vi "Unit Test Preserve wired non-serialized data (Less-Specific) True.vi"() -> ()   [LabVIEW 2019, in "Sports Unit Tests.lvclass"]
uses:
  Sports Unit Tests.lvclass
  <userlib>/Blue Origin/BlueSerialization/BlueSerializer/DeserializeOptions.ctl
  <userlib>/Blue Origin/BlueSerialization/BlueSerializer/DeserializeSlicingOptions.ctl
  <userlib>/Blue Origin/BlueSerialization/BlueSerializer/DeserializeMutationOptions.ctl
  <userlib>/Blue Origin/BlueSerialization/BlueSerializer/DeserializePreservationOptions.ctl
  <userlib>/Blue Origin/BlueSerialization/BlueSerializer/PreserveNonWiredDataOption.ctl
  Classes/The Waterboy/The Waterboy.lvclass
  C:/DSCE code/Serialization/blueserializationdemo/Test/Sports/Classes/Human/Human.lvclass
  C:/DSCE code/Serialization/blueserializationdemo/Test/Sports/Classes/Sports Player/Sports Player.lvclass
  C:/DSCE code/Serialization/blueserializationdemo/Test/Sports/Classes/Golf Player/Golf Player.lvclass
  C:/DSCE code/Serialization/blueserializationdemo/Test/Sports/Classes/Adam Sandler/Adam Sandler.lvclass
  Classes/Adam Sandler/Adam Sandler.lvclass
  Classes/Human/Human.lvclass/Human.ctl
  Classes/Sports Player/Sports Player.lvclass/Sports Player.ctl
  Classes/Golf Player/Golf Player.lvclass/Golf Player.ctl
  Classes/Adam Sandler/Adam Sandler.lvclass/Adam Sandler.ctl
  Classes/Human/Write Age (years).vi
  Classes/Human/Write alive_.vi
  Classes/Human/Write Height (ft).vi
  Classes/Human/Write Name.vi
  Classes/Sports Player/Write Earnings (dollars).vi
  Classes/Sports Player/Write Professional_.vi
  Classes/Sports Player/Write Sponsor.vi
  Classes/Golf Player/Write # holes in one.vi
  Classes/Golf Player/Write League.vi
  Classes/Golf Player/Write longest drive (ft).vi
  Classes/Adam Sandler/Write Movie Name.vi
  Classes/Adam Sandler/Write Private number.vi
  Classes/Adam Sandler/Write Secret phrase.vi
  Classes/Adam Sandler/Read Secret phrase.vi
  <vilib>/Utility/error.llb/Clear Errors.vi
  <vilib>/addons/_JKI Toolkits/Caraya/classes/Test/Define Test.vi
  <vilib>/addons/_JKI Toolkits/Caraya/classes/Assert/Assert Equal Value_Variant.vi
  <vilib>/addons/_JKI Toolkits/Caraya/classes/Assert/Assert Not Error.vi
  <vilib>/addons/_JKI Toolkits/Caraya/classes/Assert/Assert.lvclass
  <userlib>/Blue Origin/BlueSerialization/BlueSerializer/BlueSerializer.lvclass
panel:
  out "Table":string[][](table)
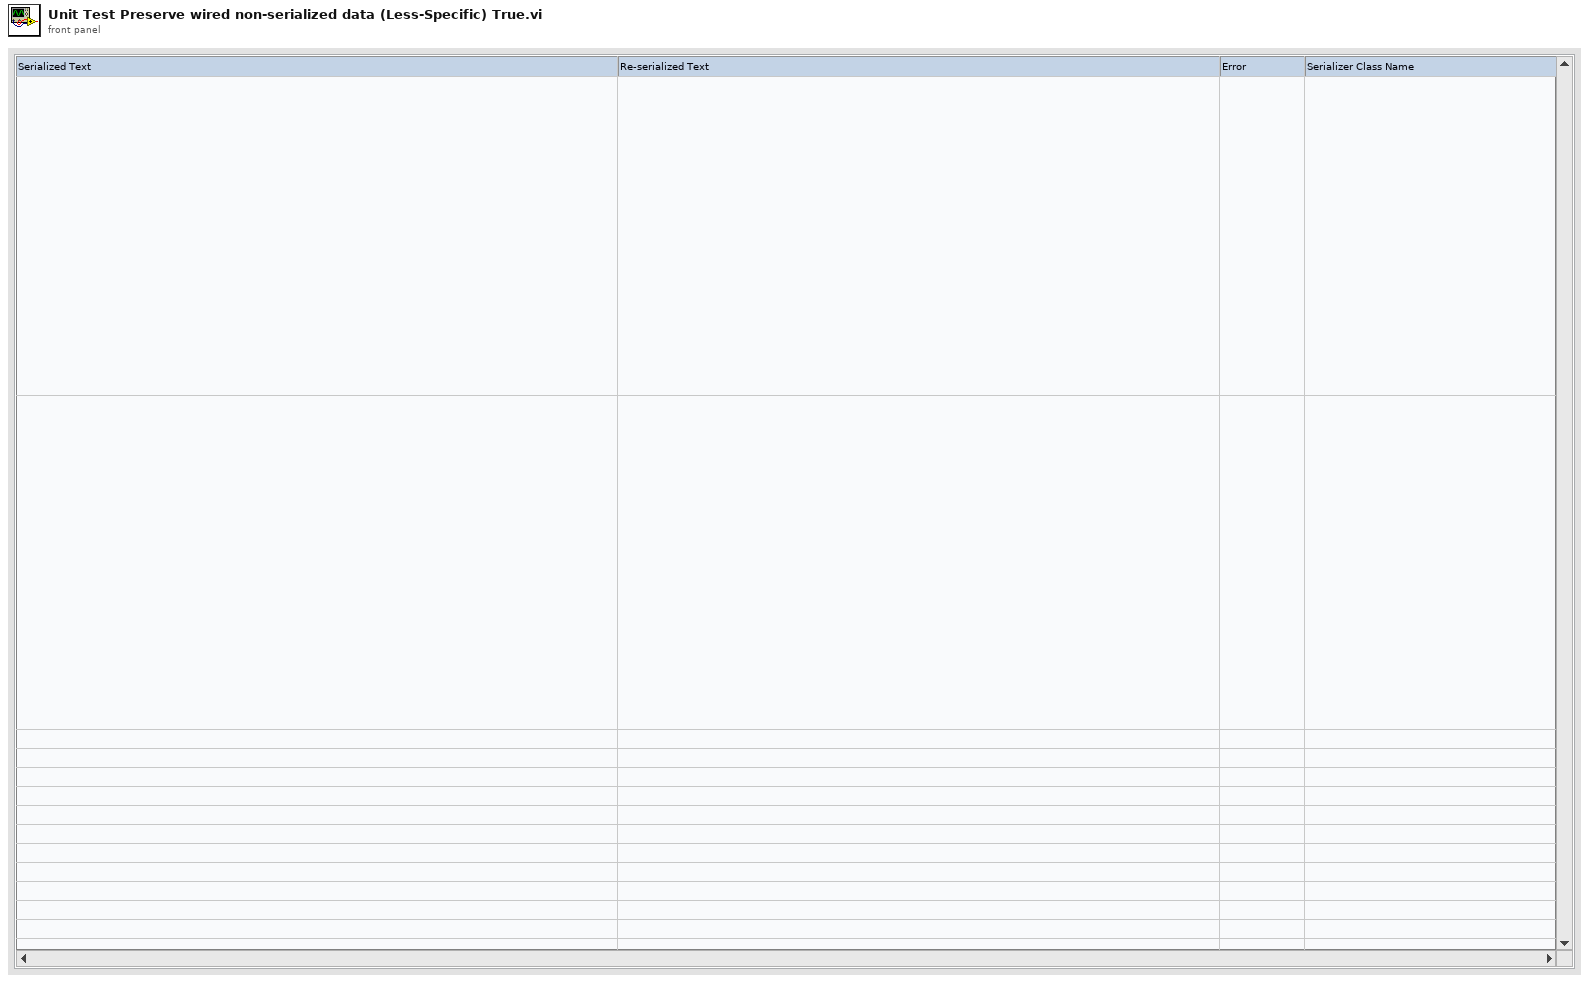
[diagram p1: front panel]
types:
  T1 = typedef "BlueSerialization.lvlib/BlueSerializer.lvclass/PreserveNonWiredDataOption.ctl" = enum16{"Don't preserve", "Preserve (error on less-specific wired types)", "Preserve (except on less-specific wired types)"}
  T2 = typedef "BlueSerialization.lvlib/BlueSerializer.lvclass/DeserializeOptions.ctl" = cluster{"deserialize non-BlueSerializable objects from hex?":bool, "expand objects on type conflict?":bool, "Slicing":T3, "Mutation Options":T4, "Preservation Options":T5}
  T3 = typedef "BlueSerialization.lvlib/BlueSerializer.lvclass/DeserializeSlicingOptions.ctl" = cluster{"slice flattened object data on error?":bool, "sliceable class names":string[]}
  T4 = typedef "BlueSerialization.lvlib/BlueSerializer.lvclass/DeserializeMutationOptions.ctl" = cluster{"error on inserted parent levels?":bool, "\terror on obsolete parent levels?":bool}
  T5 = typedef "BlueSerialization.lvlib/BlueSerializer.lvclass/DeserializePreservationOptions.ctl" = cluster{"Preserve wired serialized data?":bool, "Preserve wired non-serialized data":T1}
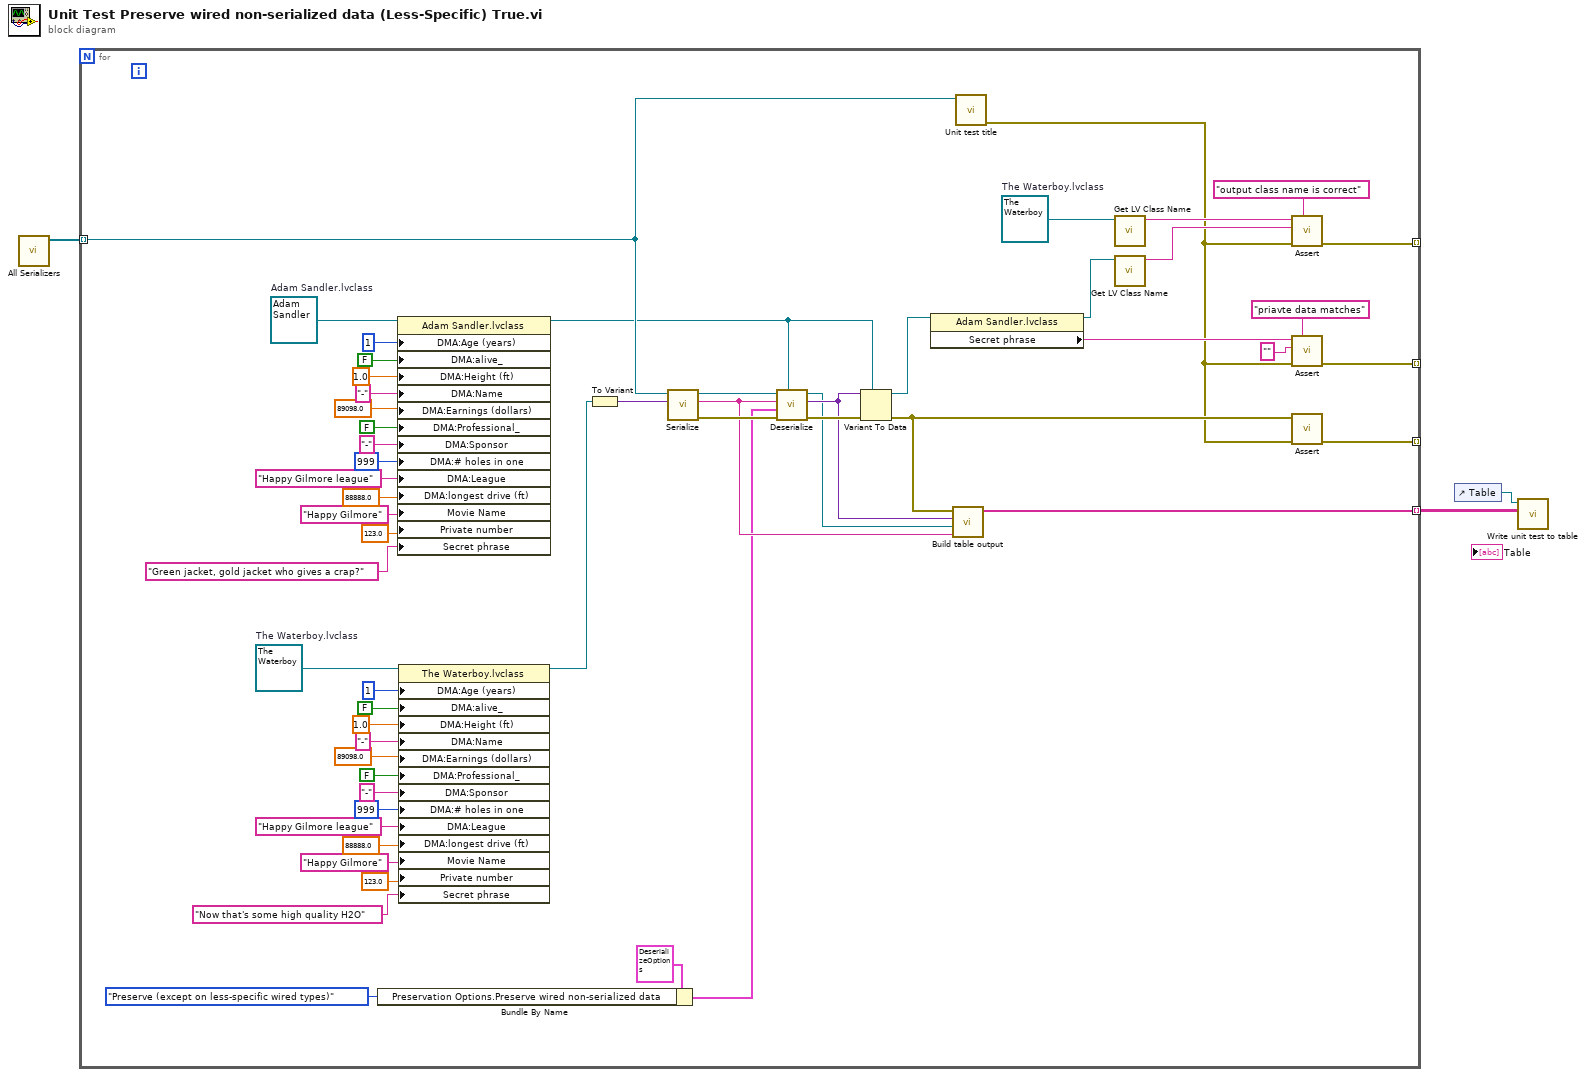
[diagram p0: block diagram]
diagram:
  n1 = call "All Serializers.vi"() -> ("All serializers"=w2:refnum<class "BlueSerializer.lvclass">[])  [unwired: 11 in]
  n2 = for {
    tunnel: w2 -> [w24] mode=indexing
    tunnel: [w45] -> _ mode=indexing
    tunnel: [w44] -> _ mode=indexing
    tunnel: [w39] -> w1 mode=indexing
    tunnel: [w28] -> _ mode=indexing
    w6 = refnum<class "The Waterboy.lvclass"> refnum  # The Waterboy.lvclass
    w7 = refnum<class "Adam Sandler.lvclass"> refnum  # Adam Sandler.lvclass
    w8 = refnum<class "The Waterboy.lvclass"> refnum  # The Waterboy.lvclass
    n3 = Bundle By Name(cluster=T2 {"deserialize non-BlueSerializable objects from hex?"=FALSE, "expand objects on type conflict?"=FALSE, "Slicing"={"slice flattened object data on error?"=FALSE, "sliceable class names"=[]}, "Mutation Options"={"error on inserted parent levels?"=FALSE, "\terror on obsolete parent levels?"=FALSE}, "Preservation Options"={"Preserve wired serialized data?"=FALSE, "Preserve wired non-serialized data"=enum."Don't preserve"}} ("Deserialize Options"), "Preservation Options.Preserve wired non-serialized data"=PreserveNonWiredDataOption."Preserve (except on less-specific wired types)") -> (w25:T2)
    n4 = property on="Property Node" class="Adam Sandler.lvclass"(reference=w7, "DMA:Age (years)"=u16 1 ("Age (years)"), "DMA:alive_"=FALSE ("alive_"), "DMA:Height (ft)"=1.0 ("Height (ft)"), "DMA:Name"="-" ("Name"), "DMA:Earnings (dollars)"=89098.0 ("Earnings (dollars)"), "DMA:Professional_"=FALSE ("Professional_"), "DMA:Sponsor"="-" ("Sponsor"), "DMA:# holes in one"=999 ("# holes in one"), "DMA:League"="Happy Gilmore league" ("League"), "DMA:longest drive (ft)"=88888.0 ("longest drive (ft)"), "Movie Name"="Happy Gilmore", "Private number"=123.0, "Secret phrase"="Green jacket, gold jacket who gives a crap?") -> (reference out=w9:refnum<class "Adam Sandler.lvclass">)  [unwired: 1 in, 1 out]
    n5 = property on="Property Node" class="The Waterboy.lvclass"(reference=w8, "DMA:Age (years)"=u16 1 ("Age (years)"), "DMA:alive_"=FALSE ("alive_"), "DMA:Height (ft)"=1.0 ("Height (ft)"), "DMA:Name"="-" ("Name"), "DMA:Earnings (dollars)"=89098.0 ("Earnings (dollars)"), "DMA:Professional_"=FALSE ("Professional_"), "DMA:Sponsor"="-" ("Sponsor"), "DMA:# holes in one"=999 ("# holes in one"), "DMA:League"="Happy Gilmore league" ("League"), "DMA:longest drive (ft)"=88888.0 ("longest drive (ft)"), "Movie Name"="Happy Gilmore", "Private number"=123.0, "Secret phrase"="Now that's some high quality H2O") -> (reference out=w10:refnum<class "The Waterboy.lvclass">)  [unwired: 1 in, 1 out]
    n6 = To Variant(anything=w10) -> (Variant=w57:variant)
    n7 = call <userlib>:"Serialize.vi"("Anything"=w57, "BlueSerializer in"=w24) -> ("error out"=w59:errorcluster, "Serialized Text"=w40:string, "BlueSerializer out"=w58:refnum<class "BlueSerializer.lvclass">)  [unwired: 7 in]
    n8 = call <userlib>:"Deserialize.vi"("Anything"=w9, "error in (no error)"=w59, "Deserialize Options"=w25, "Serialized Text"=w40, "BlueSerializer in"=w58) -> ("error out"=w56:errorcluster, "Variant"=w42:variant, "BlueSerializer out"=w41:refnum<class "BlueSerializer.lvclass">)  [unwired: 4 in]
    n9 = Variant To Data(error in=w56, type=w9, Variant=w42) -> (data=w32:refnum<class "Adam Sandler.lvclass">, error out=w43:errorcluster)
    n10 = property on="Property Node" class="Adam Sandler.lvclass"(reference=w32) -> (reference out=w31:refnum<class "Adam Sandler.lvclass">, "Secret phrase"=w30:string)  [unwired: 1 in, 1 out]
    n11 = call "Build table output.vi"("serialized text"=w40, "BlueSerializer in"=w41, "deserialized variant"=w42, "variant to data error"=w43) -> ("table output"=w39:string[])  [unwired: 7 in]
    n12 = call "Unit test title.vi"("serializer"=w24) -> ("error out"=w29:errorcluster)  [unwired: 9 in, 1 out]
    n13 = call <vilib>:"Get LV Class Name.vi"("object"=w6) -> ("class name"=w55:string)  [unwired: 9 in, 1 out]
    n14 = call <vilib>:"Get LV Class Name.vi"("object"=w31) -> ("class name"=w54:string)  [unwired: 9 in, 1 out]
    n15 = call-poly <vilib>:"Assert.vi"("Label"="output class name is correct", "error in (no error)"=w29, "Y"=w54, "X"=w55) -> ("error out"=w44:errorcluster)  [unwired: 7 in]
    n16 = call-poly <vilib>:"Assert.vi"("Label"="priavte data matches", "error in (no error)"=w29, "Y"="" ("Secret phrase"), "X"=w30) -> ("error out"=w28:errorcluster)  [unwired: 7 in]
    n17 = call-poly <vilib>:"Assert.vi"("error in (no error)"=w29, "Not Error?"=w43) -> ("error out"=w45:errorcluster)  [unwired: 9 in]
  }
  n18 = control-ref of="Table"() -> (w3:refnum<vi>)
  n19 = call "Write unit test to table.vi"("Table"=w1, "Table ref in"=w3) -> ()  [unwired: 9 in, 1 out]
